vi "Rename GObjects.vi"(8 "error in (no error)":errorcluster, 11 "ProjectItem in":refnum<class "ProjectItem.lvclass">) -> (0 "error out":errorcluster, 3 "ProjectItem out":refnum<class "ProjectItem.lvclass">)   [LabVIEW 2019, in "ProjectItem.lvclass"]
uses:
  ProjectItem.lvclass
  ProjectItem.lvclass/ProjectItem.ctl
panel:
  out "VI Names":string[](array[string])
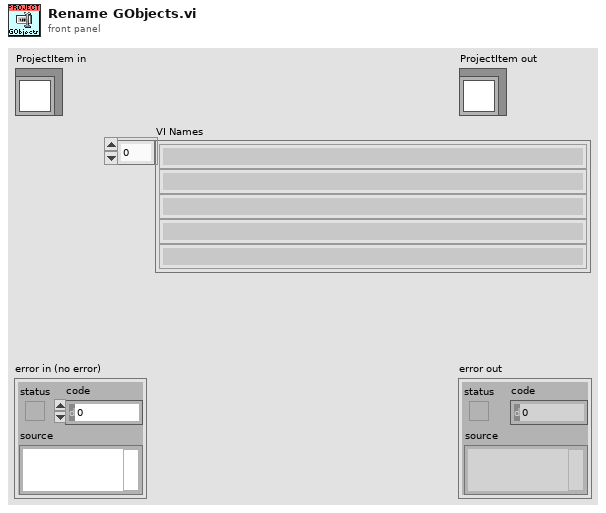
[diagram p1: front panel]
types:
  T1 = cluster{"Class":refnum<vi>, "DynamicVIs":refnum<vi>[], "StaticVIs":refnum<vi>[], "Controls":refnum<vi>[], "Name":string, "Icon":refnum<class "Icon.lvclass">, "Wire Foreground Color":u32}[]
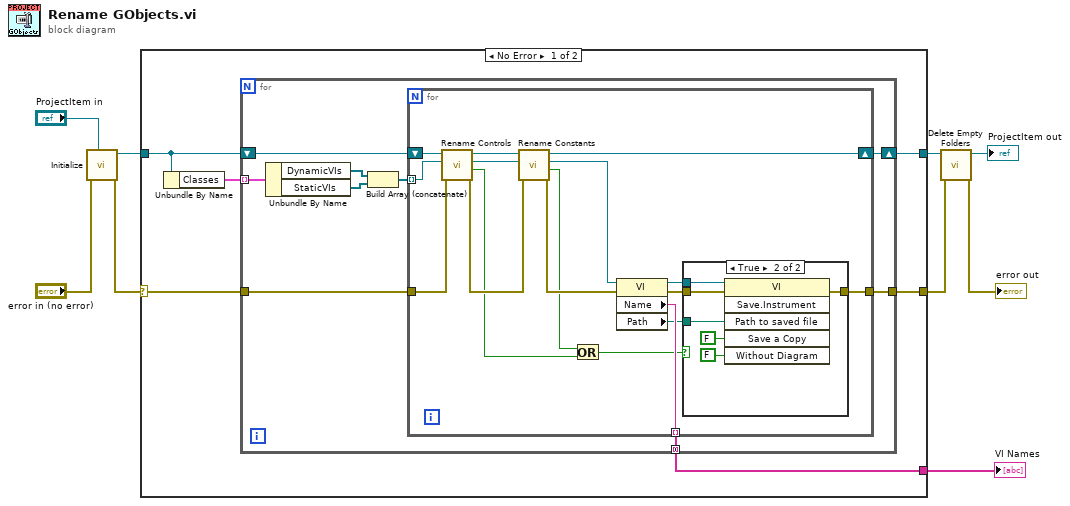
[diagram p0: block diagram]
diagram:
  n1 = call "Initialize.vi"("ProjectItem"="ProjectItem in", "error in (no error)"="error in (no error)") -> ("error out"=w6:errorcluster, "ProjectItem out"=w8:refnum<class "ProjectItem.lvclass">)  [unwired: 8 in]
  n2 = case shown="No Error" w6 {
    selector: w6 -> [w14 w50]
    tunnel: [w11 w50] -> w3
    tunnel: [w15 w49] -> w5
    tunnel: w8 -> [w12 w49]
    tunnel: [w10 _] -> w1
    frame No Error {
      n3 = Unbundle By Name(w12) -> ("Classes"=w13:T1)
      n4 = for {
        tunnel: w14 -> [w24]
        shift-right: [w23] -> w15
        shift-left: w12 -> [w22]
        tunnel: w13 -> [w21] mode=indexing
        tunnel: [w20] -> w11
        tunnel: [w19] -> w10 mode=concatenating
        n5 = Unbundle By Name(w21) -> ("DynamicVIs"=w17:refnum<vi>[], "StaticVIs"=w16:refnum<vi>[])
        n6 = Build Array (concatenate)(w17, w16) -> (w18:refnum<vi>[])
        n7 = for {
          tunnel: w24 -> [w33]
          shift-right: [w30] -> w23
          shift-left: w22 -> [w37]
          tunnel: [w25] -> w20
          tunnel: [w40] -> w19 mode=indexing
          tunnel: w18 -> [w35] mode=indexing
          n8 = call "Rename Controls.vi"("error in (no error)"=w33, "VI Reference"=w35, "ProjectItem in"=w37) -> ("error out"=w32:errorcluster, "Changed?"=w28:bool, "VI Reference out"=w34:refnum<vi>, "ProjectItem out"=w31:refnum<class "ProjectItem.lvclass">)  [unwired: 5 in]
          n9 = call "Rename Constants.vi"("error in (no error)"=w32, "VI Reference in"=w34, "ProjectItem in"=w31) -> ("error out"=w36:errorcluster, "Changed?"=w29:bool, "VI Reference out"=w26:refnum<vi>, "ProjectItem out"=w30:refnum<class "ProjectItem.lvclass">)  [unwired: 5 in]
          n10 = Or(x=w29, y=w28) -> (x .or. y?=w27:bool)
          n11 = property class="VI"(reference=w26, error in=w36) -> (reference out=w41:refnum<vi>, error out=w38:errorcluster, "Name"=w40:string, "Path"=w39:path)
          n12 = case shown="True" w27 {
            tunnel: w41 -> [_ w48]
            tunnel: w38 -> [w42 w44]
            tunnel: w39 -> [_ w45]
            tunnel: [w42 w43] -> w25
            frame False {
            }
            frame True {
              n13 = invoke class="VI" method="Save.Instrument"(reference=w48, error in=w44, "Path to saved file"=w45, "Save a Copy"=FALSE, "Without Diagram"=FALSE) -> (error out=w43:errorcluster)  [unwired: 1 in, 5 out]
            }
          }
        }
      }
    }
    frame Error {
    }
  }
  "VI Names" <- w1
  n14 = call "Delete Empty Folders.vi"("error in (no error)"=w3, "Rename in"=w5) -> ("error out"=→"error out":errorcluster, "Rename out"=→"ProjectItem out":refnum<class "ProjectItem.lvclass">)  [unwired: 8 in]
